vi "Keithley 6487 Current Read.vi"(0 "VISA resource name":refnum<visa-resource-name>, 1 "error in (no error)":errorcluster) -> (2 "VISA out":refnum<visa-resource-name>, 3 "Current (A)":dbl, 4 "error out":errorcluster)   [LabVIEW 2020]
uses:
  <vilib>/Analysis/baseanly.llb/Mean (DBL).vi
  <vilib>/Analysis/NI_AALBase.lvlib
panel:
  in  "Error procedure":string
  out "read buffer":string
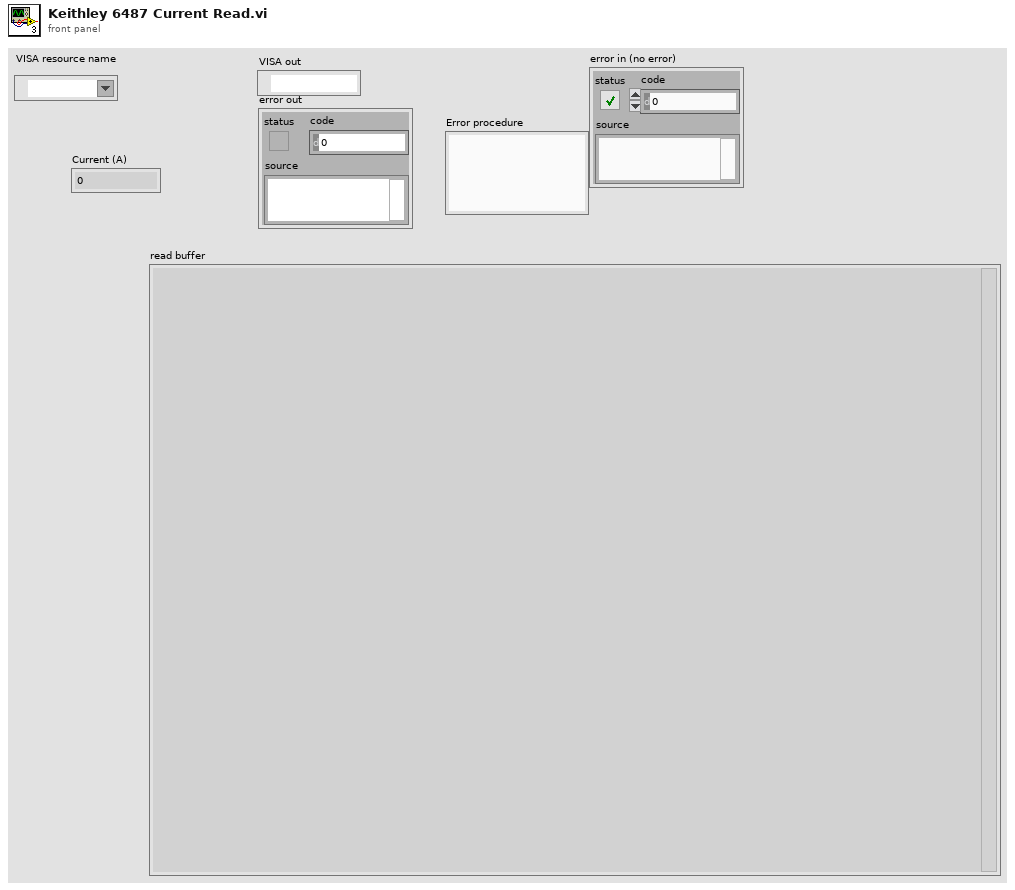
[diagram p1: front panel]
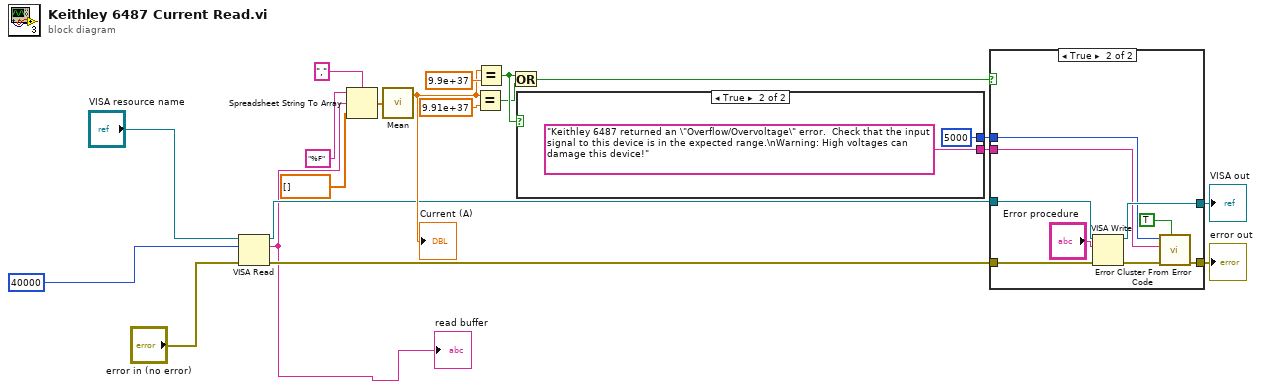
[diagram p0: block diagram]
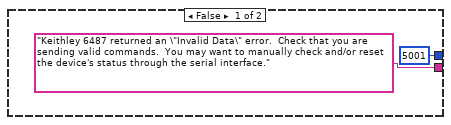
[diagram p2: hidden frame]
diagram:
  n1 = VISA Read(VISA resource name="VISA resource name", byte count=u32 40000, error in (no error)="error in (no error)") -> (VISA resource name out=w13:refnum<visa-resource-name>, read buffer=w4:string, error out=w12:errorcluster)  [unwired: 1 out]
  "read buffer" <- w4
  n2 = Spreadsheet String To Array(delimiter (Tab)=",", format string="%F", spreadsheet string=w4, array type (2D Dbl)=dbl[] [] ("Array")) -> (array=w17:dbl[])
  n3 = call-poly <vilib>:"Mean.vi"("X"=w17) -> ("mean"=w14:dbl)  [unwired: 1 out]
  "Current (A)" <- w14
  n4 = Equal?(x=w14, y=9.91e+37) -> (x = y?=w8:bool)
  n5 = Equal?(x=w14, y=9.9e+37) -> (x = y?=w9:bool)
  n6 = Or(x=w9, y=w8) -> (x .or. y?=w10:bool)
  n7 = case shown="True" w9 {
    tunnel: ["Keithley 6487 returned an \"Invalid Data\" error.  Check that you are sending valid commands.  You may want to manually check and/or reset the device's status through the serial interface." "Keithley 6487 returned an \"Overflow/Overvoltage\" error.  Check that the input signal to this device is in the expected range.\nWarning: High voltages can damage this device!"] -> w6
    tunnel: [5001 ("error code (0)") 5000 ("error code (0)")] -> w5
    frame False {
    }
    frame True {
    }
  }
  n8 = case shown="True" w10 {
    tunnel: w13 -> [w26 w35]
    tunnel: w12 -> [w25 w34]
    tunnel: [w26 w33] -> w11
    tunnel: [w25 w30] -> w7
    tunnel: w6 -> [_ w29]
    tunnel: w5 -> [_ w27]
    frame False {
    }
    frame True {
      n9 = VISA Write(VISA resource name=w35, write buffer="Error procedure", error in (no error)=w34) -> (VISA resource name out=w33:refnum<visa-resource-name>, error out=w31:errorcluster)  [unwired: 1 out]
      n10 = call <vilib>:"Error Cluster From Error Code.vi"("show call chain? (False)"=TRUE, "error in (no error)"=w31, "error message (\"\")"=w29, "error code (0)"=w27) -> ("error out"=w30:errorcluster)  [unwired: 5 in]
    }
  }
  "VISA out" <- w11
  "error out" <- w7
